vi "LVClasse_Surface Write Surface.vi"(8 "error in (no error)":errorcluster, 10 "Surface":i32, 11 "Surface in":refnum<class "Surface.lvclass">) -> (0 "error out":errorcluster, 3 "Surface out":refnum<class "Surface.lvclass">)   [LabVIEW 2020, in "Surface.lvclass"]
uses:
  Surface.lvclass
  Surface.lvclass/Surface.ctl
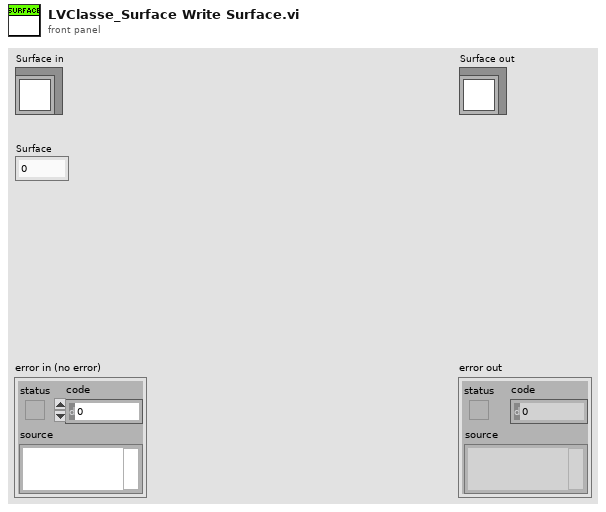
[diagram p1: front panel]
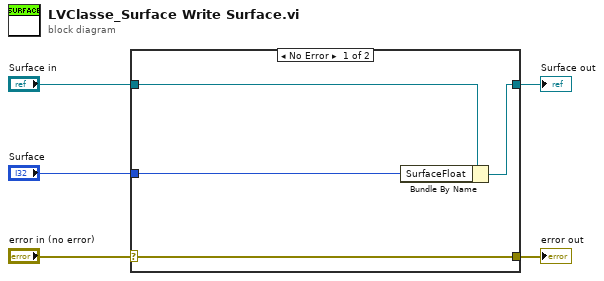
[diagram p0: block diagram]
diagram:
  n1 = case shown="No Error" "error in (no error)" {
    selector: "error in (no error)" -> [w9 w10]
    tunnel: [w9 w10] -> w4
    tunnel: [w7 w11] -> w2
    tunnel: "Surface in" -> [w8 w11]
    tunnel: "Surface" -> [w6 _]
    frame No Error {
      n2 = Bundle By Name(cluster=w8, "SurfaceFloat"=w6) -> (w7:refnum<class "Surface.lvclass">)
    }
    frame Error {
    }
  }
  "error out" <- w4
  "Surface out" <- w2
